vi "Load Single Gate Image from Becker-Hickl .sdt File.vi"(6 "Action":T1, 8 "error in (no error)":errorcluster, 10 "File Info":variant, 11 "Gate Index":i32) -> (0 "error out":errorcluster, 1 "Data 2":sgl[][](array[numeric]), 3 "Data 1":sgl[][](array[numeric]))   [LabVIEW 2021, in "Becker-Hickl Files.lvlib"]
uses:
  Becker-Hickl Files.lvlib
  AlliGator/AlliGator FLI Image Stack Action.ctl
  Becker-Hickl File Information.ctl
  Becker-Hickl File Header Structure.ctl
  Becker-Hickl Image Parameters.ctl
  Becker-Hickl TAC Parameters.ctl
  Becker-Hickl Measurement Information.ctl
  Becker-Hickl Measurement Stop Info.ctl
  Becker-Hickl FCS Measurement Info.ctl
  Becker-Hickl Additional Histogram Measurement Info.ctl
  Becker-Hickl FLIM Image Sizes.ctl
  AlliGator/AlliGator HDF5.lvlib
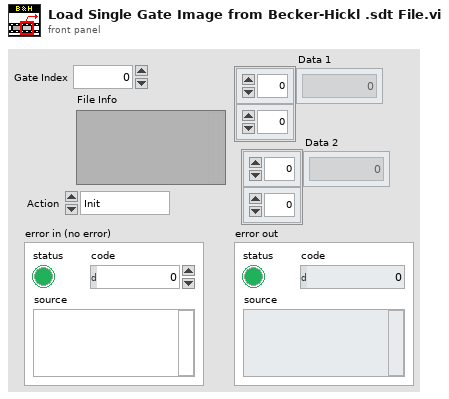
[diagram p1: front panel]
types:
  T1 = typedef "AlliGator HDF5.lvlib/AlliGator FLI Image Stack Action.ctl" = enum16{"Init", "Get Image", "Close"}
  T2 = typedef "Becker-Hickl Files.lvlib/Becker-Hickl FLIM Image Sizes.ctl" = cluster{"Image X":i32, "Image Y":i32, "ADC bins":i32}
  T3 = typedef "Becker-Hickl Files.lvlib/Becker-Hickl File Information.ctl" = cluster{"Information String":string, "File Header":T4, "Image Parameters":T5, "TAC Parameters":T6, "Measurement Information":T7, "File Path":path}
  T4 = typedef "Becker-Hickl Files.lvlib/Becker-Hickl File Header Structure.ctl" = cluster{"Revision":i16, "Info Offset":i32, "Info Length":i16, "Setup Offset":i32, "Setup Length":i16, "Data Block Offset":i32, "# Data Blocks":i16, "Data Block Length":i32, "Measurement Description Block Offset":i32, "# Measurement Description Blocks":i16, "Measurement Description Length":i16, "Header Valid":u16, "Reserved 1":u32, "Reserved 2":u16, "Checksum":u16}
  T5 = typedef "Becker-Hickl Files.lvlib/Becker-Hickl Image Parameters.ctl" = cluster{"Pixel T (s)":dbl, "Scan X":i32, "Scan Y":i32, "Image X":i32, "Image Y":i32}
  T6 = typedef "Becker-Hickl Files.lvlib/Becker-Hickl TAC Parameters.ctl" = cluster{"Frequency (Hz)":dbl, "Frequency Divider":i32, "TAC Range (s)":dbl, "TAC Gain":i32, "TAC Offset (%)":dbl, "TAC Limit Low (%)":dbl, "TAC Limit High (%)":dbl, "TAC Bin (s)":dbl, "ADC bins":i32, "Histogram Range (s)":dbl}
  T7 = typedef "Becker-Hickl Files.lvlib/Becker-Hickl Measurement Information.ctl" = cluster{"Measurement Stop Info":T8, "Measurement FCS Info":T9, "Addl Histogram Measurement Info":T10, "Creation Time":string, "Creation Date":string, "Module Serial Number":string, "Measurement Mode":i16, "CFD LL":sgl, "CFD LH":sgl, "CFD ZC":sgl, "CFD HF":sgl, "SYN ZC":sgl, "SYN FD":i16, "SYN HF":sgl, "TAC R":sgl, "TAC G":i16, "TAC OF":sgl, "TAC LL":sgl, "TAC LH":sgl, "ADC RE":i16, "EAL DE":i16, "NCX":i16, "NCY":i16, "Page":u16, "Col T":sgl, "Rep T":sgl, "Stop T":i16, "Overflow":u8, "Use Motor":i16, "Steps":u16, "Offset":sgl, "Dither":i16, "Increment":i16, "Memory Bank":i16, "Module Type":string, "SYN Th":sgl, "Dead Time Compensation":i16, "Polarity L":i16, "Polarity F":i16, "Polarity P":i16, "Line Divider":i16, "Accumulate":i16, "Flyback Y":i32, "Flyback X":i32, "Border U":i32, "Border L":i32, "Pixel Time":sgl, "Pixel Clock":i16, "Trigger":i16, "Scan X":i32, "Scan Y":i32, "Scan RX":i32, "Scan RY":i32, "FIFO Type":i16, "Exp Divider":i32, "Module Type Code":u16, "Module FPGA Version":u16, "Overflow Corr Factor":sgl, "ADC Zoom":i32, "Cycles":i32, "Image X":i32, "Image Y":i32, "Image RX":i32, "Image RY":i32, "XY Gain":i16, "Master Clock":i16, "ADC Delay":i16, "Detector Type":i16, "X Axis":i16}
  T8 = typedef "Becker-Hickl Files.lvlib/Becker-Hickl Measurement Stop Info.ctl" = cluster{"Status":u16, "Flags":u16, "Stop Time":sgl, "Current Step":i32, "Current Cycle":i32, "Current Page":i32, "Min Sync Rate":sgl, "Min CFD Rate":sgl, "Min TAC Rate":sgl, "Min ADC Rate":sgl, "Max Sync Rate":sgl, "Max CFD Rate":sgl, "Max TAC Rate":sgl, "Max ADC Rate":sgl, "Reserved 1":i32, "Reserved 2":sgl}
  T9 = typedef "Becker-Hickl Files.lvlib/Becker-Hickl FCS Measurement Info.ctl" = cluster{"Channel":u16, "FCS Decay Calc":u16, "Macrotime Resolution (0.1 ns)":u32, "Correlation Time (ms)":sgl, "# Photons":u32, "# FCS Points":i32, "End Time":sgl, "# FIFO Overflows":u16, "FCS Type":u16, "# Cross FCS Channel":u16, "Module Number":u16, "Cross FCS Module Number":u16, "Cross FCS Macrotime Resolution (0.1 ns)":u32}
  T10 = typedef "Becker-Hickl Files.lvlib/Becker-Hickl Additional Histogram Measurement Info.ctl" = cluster{"FIDA Time (ms)":sgl, "FILDA Time (ms)":sgl, "# FIDA Points":i32, "# FILDA Points":i32, "MCS Time (ms)":sgl, "# MCS Points":i32, "# Cross FCS Photons":u32, "Reserved1":i32, "Reserved2":dbl, "Reserved3":dbl}
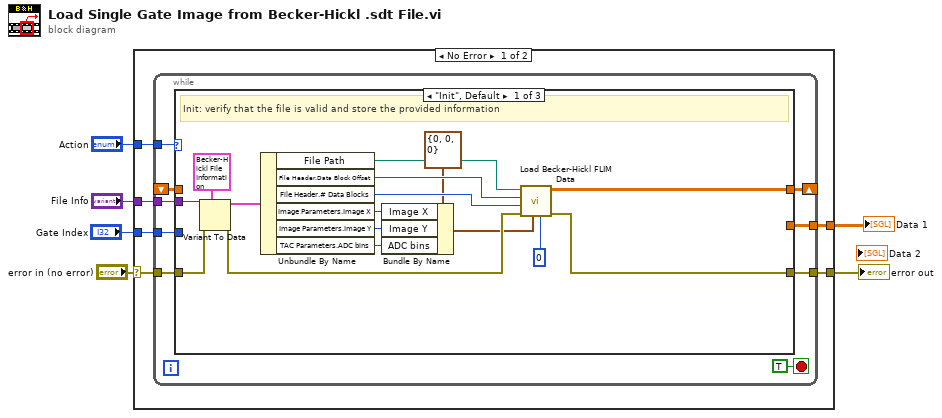
[diagram p0: block diagram]
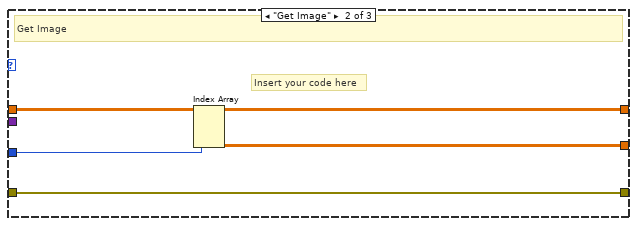
[diagram p2: hidden frame]
diagram:
  n1 = case shown="No Error" "error in (no error)" {
    selector: "error in (no error)" -> [w11 w43]
    tunnel: [w10 w43] -> w5
    tunnel: "Action" -> [w12 _]
    tunnel: "File Info" -> [w9 _]
    tunnel: "Gate Index" -> [w8 _]
    tunnel: [w7 _] -> w1
    frame No Error {
      n2 = while {
        tunnel: w12 -> [w20]
        tunnel: w11 -> [w19]
        tunnel: [w18] -> w10
        tunnel: w9 -> [w17]
        tunnel: w8 -> [w16]
        tunnel: [w15] -> w7
        shift-right: [w14] -> _
        shift-left: _ -> [w13]
        stop <- TRUE stop-if-true
        n3 = case shown="\"Init\", Default" w20 {
          tunnel: w19 -> [w36 w41 w42]
          tunnel: [w24 w41 w42] -> w18
          tunnel: w17 -> [w37 _ _]
          tunnel: w16 -> [_ w40 _]
          tunnel: [_ w39 _] -> w15
          tunnel: [w23 w38 _] -> w14
          tunnel: w13 -> [_ w38 _]
          frame "Init", Default {
            # "Init: verify that the file is valid and store the provided information"
            n4 = Variant To Data(error in=w36, type=T3 {"Information String"="", "File Header"={"Revision"=0, "Info Offset"=0, "Info Length"=0, "Setup Offset"=0, "Setup Length"=0, "Data Block Offset"=0, "# Data Blocks"=0, "Data Block Length"=0, "Measurement Description Block Offset"=0, "# Measurement Description Blocks"=0, "Measurement Description Length"=0, "Header Valid"=0, "Reserved 1"=0, "Reserved 2"=0, "Checksum"=0}, "Image Parameters"={"Pixel T (s)"=0.0, "Scan X"=0, "Scan Y"=0, "Image X"=0, "Image Y"=0}, "TAC Parameters"={"Frequency (Hz)"=0.0, "Frequency Divider"=0, "TAC Range (s)"=0.0, "TAC Gain"=0, "TAC Offset (%)"=0.0, "TAC Limit Low (%)"=0.0, "TAC Limit High (%)"=0.0, "TAC Bin (s)"=0.0, "ADC bins"=0, "Histogram Range (s)"=0.0}, "Measurement Information"={"Measurement Stop Info"={"Status"=0, "Flags"=0, "Stop Time"=0.0, "Current Step"=0, "Current Cycle"=0, "Current Page"=0, "Min Sync Rate"=0.0, "Min CFD Rate"=0.0, "Min TAC Rate"=0.0, "Min ADC Rate"=0.0, "Max Sync Rate"=0.0, "Max CFD Rate"=0.0, "Max TAC Rate"=0.0, "Max ADC Rate"=0.0, "Reserved 1"=0, "Reserved 2"=0.0}, "Measurement FCS Info"={"Channel"=0, "FCS Decay Calc"=0, "Macrotime Resolution (0.1 ns)"=0, "Correlation Time (ms)"=0.0, "# Photons"=0, "# FCS Points"=0, "End Time"=0.0, "# FIFO Overflows"=0, "FCS Type"=0, "# Cross FCS Channel"=0, "Module Number"=0, "Cross FCS Module Number"=0, "Cross FCS Macrotime Resolution (0.1 ns)"=0}, "Addl Histogram Measurement Info"={"FIDA Time (ms)"=0.0, "FILDA Time (ms)"=0.0, "# FIDA Points"=0, "# FILDA Points"=0, "MCS Time (ms)"=0.0, "# MCS Points"=0, "# Cross FCS Photons"=0, "Reserved1"=0, "Reserved2"=0.0, "Reserved3"=0.0}, "Creation Time"="", "Creation Date"="", "Module Serial Number"="", "Measurement Mode"=0, "CFD LL"=0.0, "CFD LH"=0.0, "CFD ZC"=0.0, "CFD HF"=0.0, "SYN ZC"=0.0, "SYN FD"=0, "SYN HF"=0.0, "TAC R"=0.0, "TAC G"=0, "TAC OF"=0.0, "TAC LL"=0.0, "TAC LH"=0.0, "ADC RE"=0, "EAL DE"=0, "NCX"=0, "NCY"=0, "Page"=0, "Col T"=0.0, "Rep T"=0.0, "Stop T"=0, "Overflow"=0, "Use Motor"=0, "Steps"=0, "Offset"=0.0, "Dither"=0, "Increment"=0, "Memory Bank"=0, "Module Type"="", "SYN Th"=0.0, "Dead Time Compensation"=0, "Polarity L"=0, "Polarity F"=0, "Polarity P"=0, "Line Divider"=0, "Accumulate"=0, "Flyback Y"=0, "Flyback X"=0, "Border U"=0, "Border L"=0, "Pixel Time"=0.0, "Pixel Clock"=0, "Trigger"=0, "Scan X"=0, "Scan Y"=0, "Scan RX"=0, "Scan RY"=0, "FIFO Type"=0, "Exp Divider"=0, "Module Type Code"=0, "Module FPGA Version"=0, "Overflow Corr Factor"=0.0, "ADC Zoom"=0, "Cycles"=0, "Image X"=0, "Image Y"=0, "Image RX"=0, "Image RY"=0, "XY Gain"=0, "Master Clock"=0, "ADC Delay"=0, "Detector Type"=0, "X Axis"=0}, "File Path"=path ""} ("B&H File Information"), Variant=w37) -> (data=w34:T3, error out=w30:errorcluster)
            n5 = Unbundle By Name(w34) -> ("File Path"=w33:path, "File Header.Data Block Offset"=w32:i32, "File Header.# Data Blocks"=w31:i16, "Image Parameters.Image X"=w27:i32, "Image Parameters.Image Y"=w26:i32, "TAC Parameters.ADC bins"=w25:i32)
            n6 = Bundle By Name(cluster=T2 {"Image X"=0, "Image Y"=0, "ADC bins"=0} ("Image Sizes"), "Image X"=w27, "Image Y"=w26, "ADC bins"=w25) -> (w28:T2)
            n7 = call "Load Becker-Hickl FLIM Data.vi"("Data Block Idx"=0, "Image Sizes"=w28, "error in (no error)"=w30, "# Data Blocks"=w31, "Data Block Offset"=w32, "File Path"=w33) -> ("error out"=w24:errorcluster, "Data"=w23:sgl[][][])  [unwired: 4 in]
          }
          frame "Get Image" {
            # "Insert your code here"
            # "Get Image"
            n8 = Index Array(array=w38, index (dim 2)=w40) -> (element=w39:sgl[][])  [unwired: 2 in]
          }
          frame "Close" {
            # "Close File"
          }
        }
      }
    }
    frame Error {
    }
  }
  "Data 1" <- w1
  "error out" <- w5
